vi "SysDef.Property.Get.Node.vi"(8 "error in (no error)":errorcluster, 10 "Property Name":string, 11 "nodeID":u64) -> (0 "error out":errorcluster, 1 "Value out":u64, 3 "nodeID out":u64, 4 "Found?":bool)   [LabVIEW 2015, in "Import - Export CD Config Utility.lvlib"]
uses:
  Import - Export CD Config Utility.lvlib
  <vilib>/NI Veristand/Custom Device API/Get Item Property (Dependent Node Pointer).vi
  NationalInstruments.VeriStand.SystemDefinitionAPI
  <vilib>/NI Veristand/Custom Device API/Custom Device API.lvlib
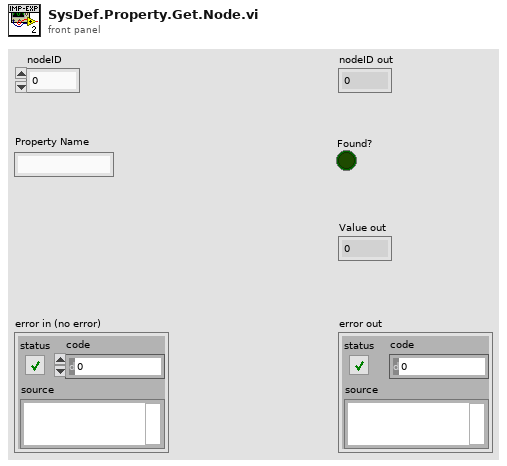
[diagram p1: front panel]
types:
  T1 = typedef "Custom Device API.lvlib/Custom Device Item Ref.ctl" = u64
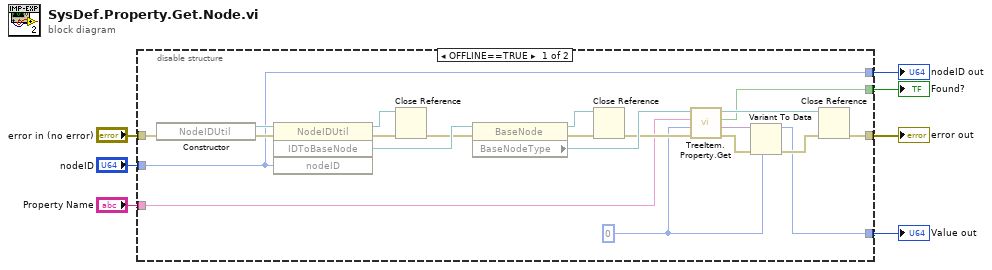
[diagram p0: block diagram]
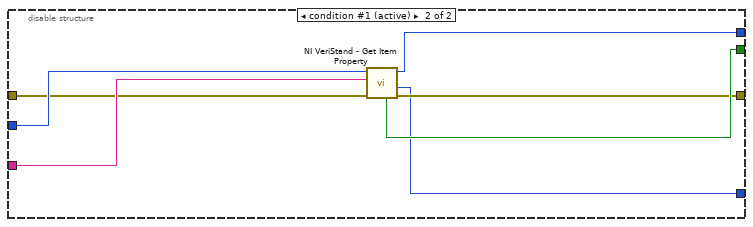
[diagram p2: hidden frame]
diagram:
  n1 = disable-structure shown="OFFLINE==TRUE" {
    disable-tunnel: "error in (no error)" -> [w21 w33]
    disable-tunnel: "nodeID" -> [w9 w34]
    disable-tunnel: [w16 w31] -> w5
    disable-tunnel: "Property Name" -> [w15 w35]
    disable-tunnel: [w11 w32] -> w3
    disable-tunnel: [w10 w29] -> w2
    disable-tunnel: [w9 w30] -> w1
    frame condition #0 {
      w8 = u64 0 ("Value out")
      n2 = constructor class="NodeIDUtil"(error in=w21) -> (reference out=w28:refnum<k24>, error out=w27:errorcluster)  [unwired: 2 in, 1 out]
      n3 = invoke class="NodeIDUtil" method="IDToBaseNode"(reference=w28, error in=w27, "nodeID"=w9) -> (reference out=w22:refnum<k24>, error out=w24:errorcluster, "IDToBaseNode"=w26:refnum<k24>)  [unwired: 1 in, 1 out]
      n4 = Close Reference(reference=w22, error in (no error)=w24) -> (error out=w23:errorcluster)
      n5 = property class="BaseNode"(reference=w26, error in=w23) -> (reference out=w20:refnum<k24>, error out=w19:errorcluster, "BaseNodeType"=w25:refnum<k24>)
      n6 = Close Reference(reference=w20, error in (no error)=w19) -> (error out=w18:errorcluster)
      n7 = call "TreeItem.Property.Get.vi"("error in (no error)"=w18, "Default Value"=w8, "Property Name"=w15, "Basenode"=w25) -> ("error out"=w13:errorcluster, "Variant"=w14:variant, "Found?"=w11:bool, "Basenode"=w17:refnum<k24>)  [unwired: 4 in]
      n8 = Variant To Data(error in=w13, type=w8, Variant=w14) -> (data=w10:u64, error out=w12:errorcluster)
      n9 = Close Reference(reference=w17, error in (no error)=w12) -> (error out=w16:errorcluster)
    }
    frame condition #1 (active) {
      n10 = call-poly <vilib>:"NI VeriStand - Get Item Property.vi"("error in (no error)"=w33, "Property Name"=w35, "Item Ref in"=w34) -> ("error out"=w31:errorcluster, "Dependent Node Ref"=w29:T1, "Item Ref out"=w30:T1, "Found"=w32:bool)  [unwired: 5 in]
    }
  }
  "nodeID out" <- w1
  "error out" <- w5
  "Value out" <- w2
  "Found?" <- w3
